vi "LVDimInterface.dic_info_service_queue.vi"(1 "serviceName":string, 2 "queueRef":T2, 3 "timeout [s]":i32=10, 4 "serviceType":T1=4 items=["ONCE_ONLY"=1, "TIMED"=2, "MONITORED"=4], 5 "error in (no error)":errorcluster, 7 "stamped":bool=TRUE) -> (14 "callBackID":i32, 19 "error out":errorcluster)   [LabVIEW 2013, in "LVDimInterface.lvlib"]
doc: "Registers a message queue to a DIM service. The data received by DIM will be inserted as a new element into the message queue. If no longer used, a registered event should be unregistered using \"release service\".\n\nHistory: 16-DEC-2005, Dietrich Beck\n\nCopyright (C)\nGesellschaft für Schwerionenforschung, GSI\nPlanckstr. 1\n64291 Darmstadt\nGermany\n\nContact: D.Beck@gsi.de \n\nThis program is free software; you can redistribute it and/or modify it under the terms of the \nGNU General Public License as published by the Free Software Foundation; either version 2 of the license, or (at your option) any later version.\n\nThis program is distributed in the hope that it will be useful, but WITHOUT ANY WARRANTY; without even the implied warranty of MERCHANTABILITY or FITNESS FOR A PARTICULAR PURPOSE. See the GNU General License for more details (http://www.gnu.org).\n\nGesellschaft für Schwerionenforschung, GSI\nPlanckstr. 1, 64291 Darmstadt, Germany\nFor all questions and ideas contact D. Beck.\nLast update: 16-DEC-2005"
uses:
  LVDimInterface.lvlib
  LVDimInterface.queue type.ctl
  LVDimInterface.dim service type.ctl
  bin/libDimWrapper.dll
  C/GPL/Projects/DimLVEvent/bin/libDimWrapper.so
  C/GPL/Projects/DimLVEvent/bin/libDimWrapperSPL.dll
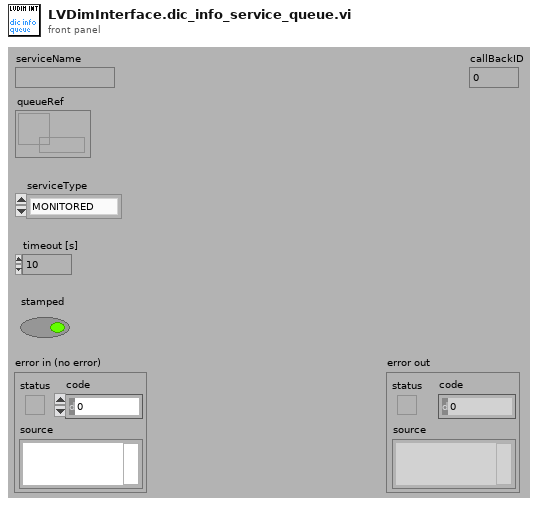
[diagram p1: front panel]
types:
  T1 = typedef "LVDimInterface.lvlib/LVDimInterface.dim service type.ctl" = u16
  T2 = typedef "LVDimInterface.lvlib/LVDimInterface.queue type.ctl" = refnum<queue>
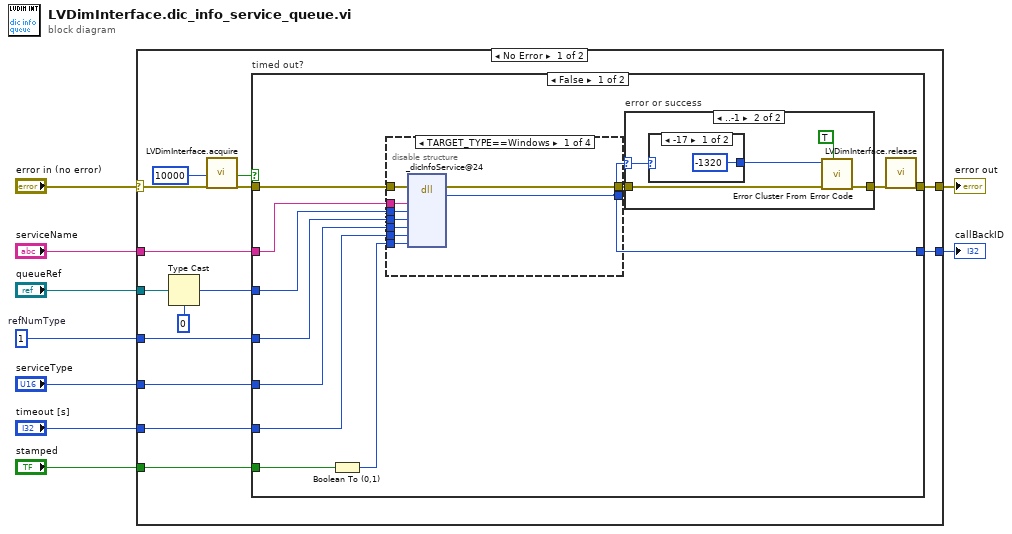
[diagram p0: block diagram]
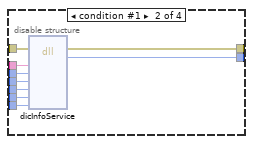
[diagram p2: hidden frame]
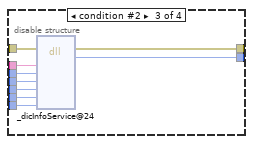
[diagram p3: hidden frame]
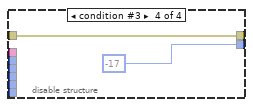
[diagram p4: hidden frame]
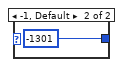
[diagram p6: hidden frame]
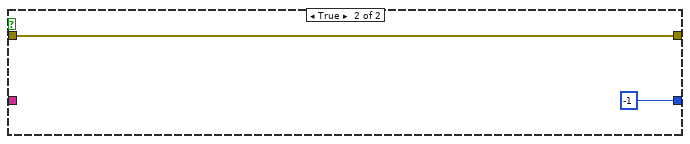
[diagram p7: hidden frame]
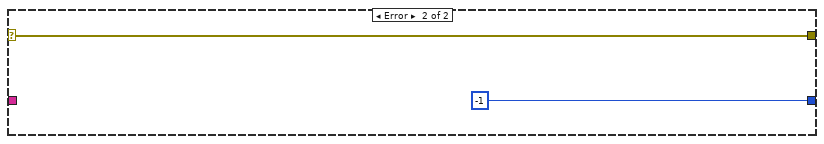
[diagram p8: hidden frame]
diagram:
  w8 = 1  # refNumType
  n1 = case shown="No Error" "error in (no error)" {
    selector: "error in (no error)" -> [w10 w76]
    tunnel: "serviceName" -> [w23 _]
    tunnel: w8 -> [w22 _]
    tunnel: "serviceType" -> [w21 _]
    tunnel: "timeout [s]" -> [w20 _]
    tunnel: [w18 -1 ("callBackID")] -> w5
    tunnel: [w19 w76] -> w3
    tunnel: "stamped" -> [w17 _]
    tunnel: "queueRef" -> [w16 _]
    frame No Error {
      n2 = Type Cast(type=u32 0, x=w16) -> (*(type *) &x=w14:u32)
      n3 = call "LVDimInterface.acquire.vi"("ms timeout (10000)"=10000 ("ms timeout (-1)"), "error in (no error)"=w10) -> ("timed out"=w12:bool, "error out"=w11:errorcluster)  [unwired: 16 in]
      n4 = case "timed out?" shown="False" w12 {
        tunnel: w23 -> [w35 _]
        tunnel: w22 -> [w34 _]
        tunnel: w21 -> [w33 _]
        tunnel: w20 -> [w32 _]
        tunnel: [w24 w73] -> w19
        tunnel: [w31 -1 ("callBackID")] -> w18
        tunnel: w17 -> [w30 _]
        tunnel: w14 -> [w28 _]
        tunnel: w11 -> [w27 w73]
        frame False {
          n5 = Boolean To (0,1)(Boolean=w30) -> (0, 1=w29:i16)
          n6 = disable-structure "Conditional Disable Structure" shown="TARGET_TYPE==Windows" {
            disable-tunnel: w35 -> [w44 w53 w62 _]
            disable-tunnel: w34 -> [w43 w52 w61 _]
            disable-tunnel: w33 -> [w42 w51 w60 _]
            disable-tunnel: w32 -> [w41 w50 w59 _]
            disable-tunnel: [w40 w49 w58 -17 ("callBackID")] -> w31
            disable-tunnel: w29 -> [w39 w48 w57 _]
            disable-tunnel: w28 -> [w38 w47 w56 _]
            disable-tunnel: w27 -> [w37 w46 w55 w63]
            disable-tunnel: [w36 w45 w54 w63] -> w26
            frame condition #0 (active) {
              n7 = dll-call lib="C:/User/Brand/LVP/Submodules/DimLVEvent/bin/libDimWrapper.dll" fn="_dicInfoService@24"(error in=w37, "serviceName"=w44, "refNum"=w38, "refNumType"=w43, "serviceType"=w42, "timeout"=w41, "stamped"=w39) -> (error out=w36:errorcluster, "callBackID"=w40:i32)  [unwired: 8 in, 1 out]
            }
            frame condition #1 {
              n8 = dll-call lib="F:/LVSCC/C/GPL/Projects/DimLVEvent/bin/libDimWrapper.so" fn="dicInfoService" label="libDimWrapper.dll:_dicInfoService@24"(error in=w46, "serviceName"=w53, "refNum"=w47, "refNumType"=w52, "serviceType"=w51, "timeout"=w50, "stamped"=w48) -> (error out=w45:errorcluster, "callBackID"=w49:i32)  [unwired: 8 in, 1 out]
            }
            frame condition #2 {
              n9 = dll-call lib="C:/User/Brand/SVN/C/GPL/Projects/DimLVEvent/bin/libDimWrapperSPL.dll" fn="_dicInfoService@24"(error in=w55, "serviceName"=w62, "refNum"=w56, "refNumType"=w61, "serviceType"=w60, "timeout"=w59, "stamped"=w57) -> (error out=w54:errorcluster, "callBackID"=w58:i32)  [unwired: 8 in, 1 out]
            }
            frame condition #3 {
            }
          }
          n10 = case "error or success" shown="..-1" w31 {
            selector: w31 -> [_ w70]
            tunnel: w26 -> [w65 w68]
            tunnel: [w65 w69] -> w25
            frame 0, Default {
            }
            frame ..-1 {
              n11 = case shown="-17" w70 {
                tunnel: [-1320 ("code") -1301 ("code")] -> w66
                frame -17 {
                }
                frame -1, Default {
                }
              }
              n12 = call <vilib>:"Error Cluster From Error Code.vi"("show call chain? (False)"=TRUE ("status"), "error in (no error)"=w68, "error code (0)"=w66) -> ("error out"=w69:errorcluster)  [unwired: 6 in]
            }
          }
          n13 = call "LVDimInterface.release.vi"("error in (no error)"=w25) -> ("error out"=w24:errorcluster)  [unwired: 18 in]
        }
        frame True {
        }
      }
    }
    frame Error {
    }
  }
  "callBackID" <- w5
  "error out" <- w3
